vi "题目4.vi"() -> ()   [LabVIEW 2017]
uses:
  <vilib>/Analysis/2dsp.llb/Real FFT.vi
  <vilib>/Analysis/NI_AALPro.lvlib
  <vilib>/measure/NI_MABase.lvlib
panel:
  in  "sampling info":cluster{"Fs":dbl, "#s":dbl}={"Fs"=1000.0, "#s"=1000.0} caption="采样信息" {"Fs" format="%.2p"}
  in  "amplitude 3":dbl=1.0 caption="幅值3" format="%0.2p"
  in  "frequency 3":dbl=10.0 caption="频率3" format="%0.2p"
  in  "amplitude 2":dbl=1.0 caption="幅值2" format="%0.2p"
  in  "frequency 2":dbl=10.0 caption="频率2" format="%0.2p"
  in  "amplitude":dbl=1.0 caption="幅值1" format="%0.2p"
  in  "frequency":dbl=10.0 caption="频率1" format="%0.2p"
  out "频域信号":dbl[](graph)
  out "时域信号":dbl[](graph)
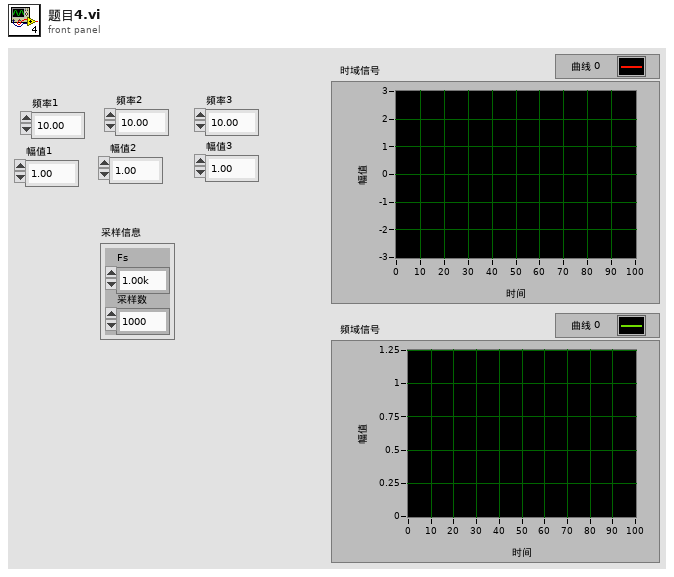
[diagram p1: front panel]
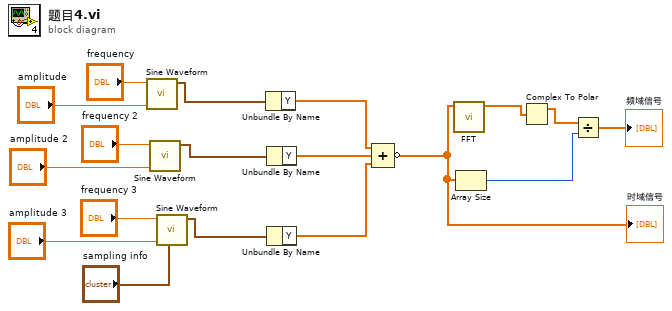
[diagram p0: block diagram]
diagram:
  n1 = call <vilib>:"Sine Waveform.vi"("amplitude"="amplitude", "frequency"="frequency") -> ("signal out"=w8:waveform(dbl))  [unwired: 8 in, 1 out]
  n2 = call <vilib>:"Sine Waveform.vi"("amplitude"="amplitude 2", "frequency"="frequency 2") -> ("signal out"=w7:waveform(dbl))  [unwired: 8 in, 1 out]
  n3 = call <vilib>:"Sine Waveform.vi"("sampling info"="sampling info", "amplitude"="amplitude 3", "frequency"="frequency 3") -> ("signal out"=w6:waveform(dbl))  [unwired: 7 in, 1 out]
  n4 = Unbundle By Name(w8) -> ("Y"=w5:dbl[])
  n5 = Unbundle By Name(w7) -> ("Y"=w4:dbl[])
  n6 = Unbundle By Name(w6) -> ("Y"=w3:dbl[])
  n7 = Compound Arithmetic op=ADD(w5, w4, w3) -> (invert w2:dbl[])
  "时域信号" <- w2
  n8 = call-poly <vilib>:"FFT.vi"("X"=w2) -> ("FFT {X}"=w16:cdb[])  [unwired: 9 in, 1 out]
  n9 = Array Size(array=w2) -> (size(s)=w17:i32)
  n10 = Complex To Polar(r * e^(i*theta)=w16) -> (r=w18:dbl[])  [unwired: 1 out]
  n11 = Divide(x=w18, y=w17) -> (x/y=→"频域信号":dbl[])
